vi "Build Grid and Rock List.vi"(11 "text data":string) -> (0 "Rock Lines":cluster{"Array":u32[][]}[](array[cluster]), 1 "Column Offset":i32, 3 "Grig":T1[][](array[typedef]))   [LabVIEW 2020]
uses:
  RB ENUM_Space ID.ctl
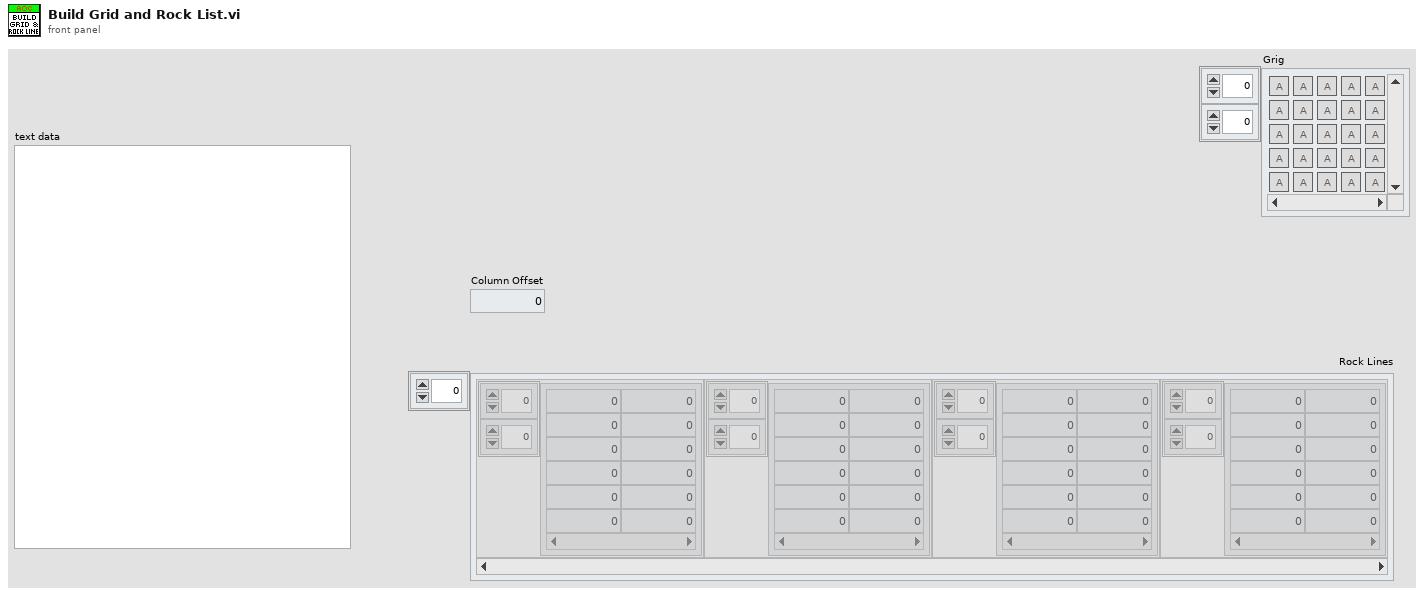
[diagram p1: front panel]
types:
  T1 = typedef "RB ENUM_Space ID.ctl" = enum32{"Air", "Sand", "Rock", "Start", "Abyss"}
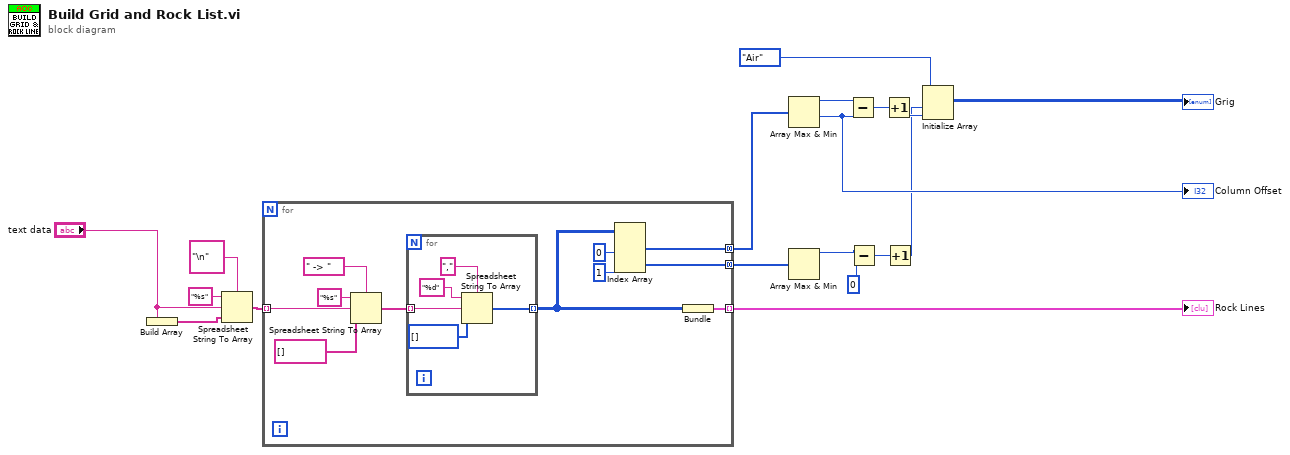
[diagram p0: block diagram]
diagram:
  n1 = Build Array("text data") -> (w1:string[])
  n2 = Spreadsheet String To Array(delimiter (Tab)="\n", format string="%s", spreadsheet string="text data", array type (2D Dbl)=w1) -> (array=w4:string[])
  n3 = for {
    tunnel: w4 -> [w29] mode=indexing
    tunnel: [w24] -> w16 mode=indexing
    tunnel: [w20] -> w6 mode=concatenating
    tunnel: [w19] -> w5 mode=concatenating
    n4 = Spreadsheet String To Array(delimiter (Tab)=" -> ", format string="%s", spreadsheet string=w29, array type (2D Dbl)=string[] []) -> (array=w25:string[])
    n5 = for {
      tunnel: w25 -> [w34] mode=indexing
      tunnel: [w30] -> w23 mode=indexing
      n6 = Spreadsheet String To Array(delimiter (Tab)=",", format string="%d", spreadsheet string=w34, array type (2D Dbl)=i32[] []) -> (array=w30:i32[])
    }
    n7 = Index Array(array=w23, index (col) #1=0 ("disabled index (col)"), index (col) #2=1 ("index (col)")) -> (element #1=w19:i32[], element #2=w20:i32[])  [unwired: 2 in]
    n8 = Bundle(w23) -> (w24:cluster{i32[][]})  [unwired: 1 in]
  }
  "Rock Lines" <- w16
  n9 = Array Max & Min(array=w5) -> (max value=w7:i32, min value=w17:i32)  [unwired: 2 out]
  "Column Offset" <- w17
  n10 = Array Max & Min(array=w6) -> (max value=w10:i32)  [unwired: 3 out]
  n11 = Subtract(x=w7, y=w17) -> (x-y=w8:i32)
  n12 = Subtract(x=w10, y=0) -> (x-y=w9:i32)
  n13 = Increment(x=w8) -> (x+1=w15:i32)
  n14 = Increment(x=w9) -> (x+1=w14:i32)
  n15 = Initialize Array(RB_ENUM_Space_ID."Air" ("Space"), w14, w15) -> (→"Grig":T1[][])
